vi "输入分辨率计算-EV05.vi"(7 "1字节?":bool, 8 "数值 2":dbl, 9 "数值":dbl, 10 "偏移量":dbl, 11 "分辨率":dbl) -> (0 "低字节 2":dbl, 1 "高字节 2":dbl, 2 "低字节":dbl, 3 "高字节1":dbl)   [LabVIEW 2013]
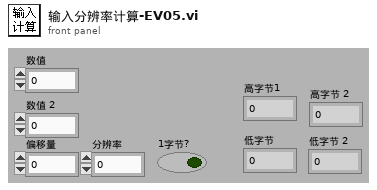
[diagram p1: front panel]
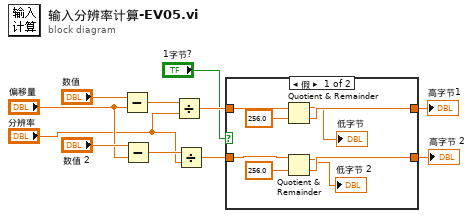
[diagram p0: block diagram]
diagram:
  n1 = Subtract(x="数值", y="偏移量") -> (x-y=w8:dbl)
  n2 = Subtract(x="数值 2", y="偏移量") -> (x-y=w7:dbl)
  n3 = Divide(x=w8, y="分辨率") -> (x/y=w5:dbl)
  n4 = Divide(x=w7, y="分辨率") -> (x/y=w4:dbl)
  n5 = case shown="假" "1字节?" {
    tunnel: w5 -> [w19 w21]
    tunnel: w4 -> [w16 w20]
    tunnel: [w15 w21] -> w2
    tunnel: [w14 w20] -> w1
    frame False {
      n6 = Quotient & Remainder(x=w19, y=256.0) -> (x-y*floor(x/y)=→"低字节":dbl, floor(x/y)=w15:dbl)
      n7 = Quotient & Remainder(x=w16, y=256.0) -> (x-y*floor(x/y)=→"低字节 2":dbl, floor(x/y)=w14:dbl)
    }
    frame True {
    }
  }
  "高字节1" <- w2
  "高字节 2" <- w1
